vi "Gyro Pose Update Loop.vi"   [LabVIEW 2017]
uses:
  <vilib>/Platform/TimedLoop/XDataNode/timing_clust.ctl
  <vilib>/Platform/TimedLoop/XDataNode/nitl_modes.ctl
  <vilib>/Platform/TimedLoop/XDataNode/wakeup.ctl
  gyro/Gyro Globals.vi
  Control Globals.vi
  <vilib>/Platform/TimedLoop/XDataNode/XDataNode.xnode
  <vilib>/Platform/TimedLoop/XDataNode/XDNodeRunTimeDep.lvlib
types:
  T1 = typedef "XDNodeRunTimeDep.lvlib/timing_clust.ctl" = cluster{"Expected End [f-1]":u64, "Actual End [f-1]":u64, "Finished Late? [f-1]":bool, "Expected End [i-1]":u64, "Actual End [i-1]":u64, "Finished Late? [i-1]":bool, "Expected Start [i]":u64, "Actual Start [i]":u64, "Expected Start [f]":u64, "Actual Start [f]":u64, "Source Name":string, "Structure Name":string, "Period":i64, "Deadline":i64, "Offset":i64, "Start":i64, "Priority":i32, "Timeout":i32, "Mode":T2, "Wakeup Reason":T3, "Error":errorcluster, "Source Type":string, "Secondary Source Type":string, "Global End Time":u64, "Global Start Time":u64, "Frame Duration":u64, "Iteration Duration":u64, "Assigned CPU":i32, "I/O Scan Engine Mode":u32}
  T2 = typedef "XDNodeRunTimeDep.lvlib/nitl_modes.ctl" = enum32{"No Change", "Process missed periods, maintain original phase", "Discard missed periods, maintain original phase", "Process missed periods, ignore original phase", "Discard missed periods, ignore original phase"}
  T3 = typedef "XDNodeRunTimeDep.lvlib/wakeup.ctl" = enum32{"Normal", "Aborted", "Asynchronous wakeup", "Timing source error", "Timed loop error", "Timeout"}
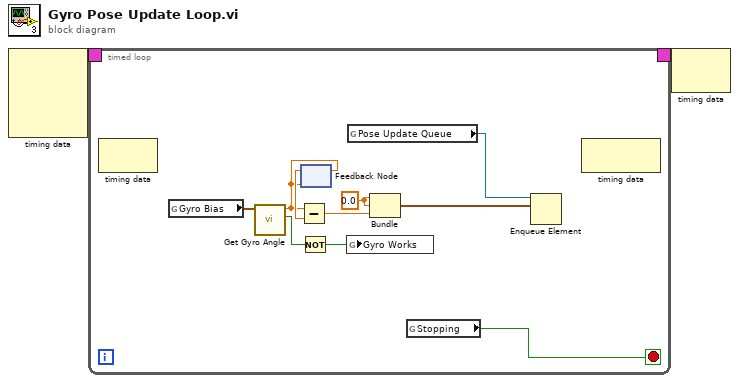
[diagram p0: block diagram]
diagram:
  n1 = node-c288() -> (w2:T1)  [unwired: 4 in]
  n2 = timed-loop {
    timing: w2 -> [_]
    timing-out: [_] -> w1
    stop <- w3 stop-if-true
    w8 = 0.0 ("x-y")
    n3 = node-c288() -> ()  [unwired: 1 in, 1 out]
    n4 = global read "Gyro Globals.vi" "Gyro Bias"() -> (w6:cluster{"X":dbl, "Y":dbl, "Z":dbl})
    n5 = call "Get Gyro Angle.vi"("Gyro bias"=w6) -> ("GYRO IS FUCKED"=w7:bool, "Z Rotation (rads)"=w11:dbl)  [unwired: 9 in]
    n6 = Not(x=w7) -> (.not. x?=w5:bool)
    n7 = feedback-in #1(w11) -> ()
    n8 = feedback #1(w11) -> (w12:dbl)
    n9 = Subtract(x=w11, y=w12) -> (x-y=w10:dbl)
    n10 = global write "Control Globals.vi" "Gyro Works"(w5) -> ()
    n11 = global read "Control Globals.vi" "Pose Update Queue"() -> (w4:refnum<queue>)
    n12 = Bundle("x-y"=w8, "x-y"=w8, w10) -> (w9:cluster{"x-y":dbl, "x-y":dbl, dbl})  [unwired: 1 in]
    n13 = global read "Control Globals.vi" "Stopping"() -> (w3:bool)
    n14 = Enqueue Element(queue=w4, element=w9) -> ()  [unwired: 2 in, 3 out]
    n15 = node-c288() -> ()  [unwired: 1 in, 1 out]
  }
  n16 = node-c288(w1) -> ()  [unwired: 1 out]
